vi "Create Evals.vi"(8 "error in (no error)":errorcluster, 10 "Step In":refnum<k7>, 11 "DCLeakage in":refnum<class "DCLeakage.lvclass">=refnum) -> (0 "error out":errorcluster, 2 "Step Out":refnum<k7>, 3 "DCLeakage out":refnum<class "DCLeakage.lvclass">)   [LabVIEW 2018, in "DCLeakage.lvlib" / "DCLeakage.lvclass"]
uses:
  DCLeakage.lvclass
  Plugins/SeqAuto Evaluations.lvlibp/DC Evaluations/DCLeakage/DCLeakage.lvclass
  Plugins/TestStand API Tools (TSAT).lvlibp/Step Actions/TSAT Step Actions.lvlib
  Plugins/Test Number and Bin Generator.lvlibp/Test Number and Bin Generator/Test Number and Bin Generator.lvclass
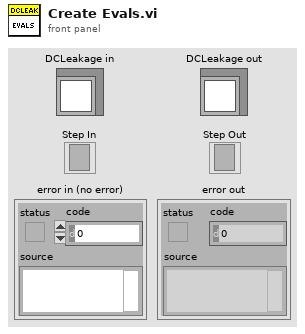
[diagram p1: front panel]
types:
  T1 = typedef "TestStand API Tools (TSAT).lvlibp/TSAT Evaluation Actions.lvlib/TSAT Evaluation.ctl" = cluster{"Test Name":string, "Pin":string, "Units":string, "SI Scaling":T2, "Test Number":i32, "Published Data Id":string, "Low Limit":dbl, "High Limit":dbl, "Export Data Location":string, "Software Bin":i64, "Evaluation Type":T3, "Test Data Source":string}
  T2 = typedef "TestStand API Tools (TSAT).lvlibp/TSAT Evaluation Actions.lvlib/TSAT Eval SI Unit Scaling.ctl" = i16
  T3 = typedef "TestStand API Tools (TSAT).lvlibp/TSAT Evaluation Actions.lvlib/TSAT Evaluation Type.ctl" = enum16{"Numeric Limit", "Pass/Fail", "None"}
  T4 = typedef "Test Number and Bin Generator.lvlibp/Test Number and Bin Generator.lvclass/Session Handle.ctl" = refnum<data-value>
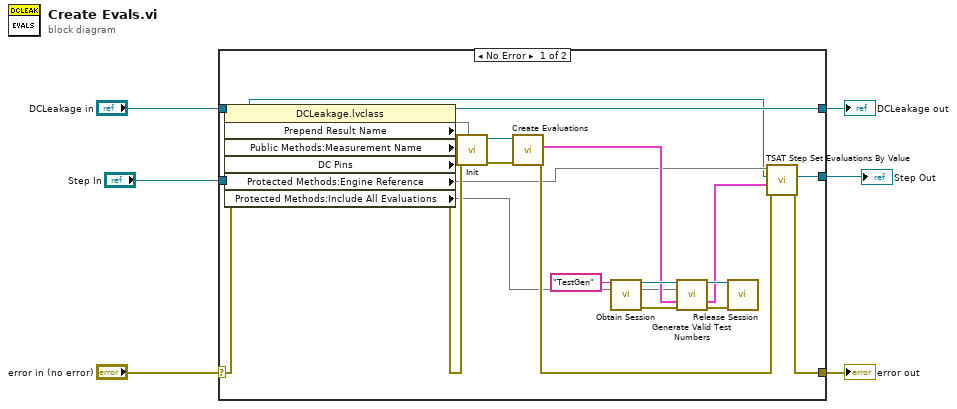
[diagram p0: block diagram]
diagram:
  n1 = case shown="No Error" "error in (no error)" {
    selector: "error in (no error)" -> [w28 w31]
    tunnel: [w13 w31] -> w5
    tunnel: [w26 w30] -> w3
    tunnel: "DCLeakage in" -> [w27 w30]
    tunnel: "Step In" -> [w11 w29]
    tunnel: [w10 w29] -> w1
    frame No Error {
      n2 = property class="DCLeakage.lvclass"(reference=w27, error in=w28) -> (reference out=w26:refnum<class "DCLeakage.lvclass">, error out=w24:errorcluster, "Prepend Result Name"=w7, "Public Methods:Measurement Name"=w8, "DC Pins"=w25, "Protected Methods:Engine Reference"=w12, "Protected Methods:Include All Evaluations"=w9)
      n3 = call "Init.vi"("Prepend Result Name"=w7, "error in (no error)"=w24, "DC Pins"=w25, "Measurement Name"=w8) -> ("error out"=w22:errorcluster, "DCLeakage out"=w23:refnum<class "DCLeakage.lvclass">)  [unwired: 6 in]
      n4 = call-dynamic "Create Evaluations.vi"("error in (no error)"=w22, "IEvaluation in"=w23) -> ("error out"=w14:errorcluster, "Evaluations Out"=w16:T1[])  [unwired: 7 in, 1 out]
      n5 = call "Obtain Session.vi"("Session  Name ()"="TestGen") -> ("Session Handle"=w21:T4, "error out"=w18:errorcluster)  [unwired: 13 in]
      n6 = call "Generate Valid Test Numbers.vi"("Session Handle in"=w21, "Include All Evaluations?"=w9, "Evaluations In"=w16, "error in (no error)"=w18) -> ("Session Handle out"=w20:T4, "Evaluations Out"=w15:T1[], "error out"=w19:errorcluster)  [unwired: 9 in]
      n7 = call "Release Session.vi"("Session Handle"=w20, "error in (no error)"=w19) -> ()  [unwired: 13 in, 1 out]
      n8 = call "TSAT Step Set Evaluations By Value.vi"("Error In"=w14, "Evaluation Data"=w15, "Step In"=w11, "Engine In"=w12) -> ("Error Out"=w13:errorcluster, "Step Out"=w10:refnum<k7>)  [unwired: 5 in, 1 out]
    }
    frame Error {
    }
  }
  "error out" <- w5
  "DCLeakage out" <- w3
  "Step Out" <- w1
